vi "Main Loop.vi"(8 "error in (no error)":errorcluster, 10 "Chart Notifier":refnum<notifier>, 11 "Message Queues":T1) -> (0 "error out":errorcluster)   [LabVIEW 2018, in "Pump Module.lvlib" / "Pump Module Engine.lvlib"]
uses:
  Pump Module Engine.lvlib
  All Message Queues.ctl
  support/Message Queue/Message Cluster.ctl
  State Cluster.ctl
  State Enum.ctl
  Pump Module Settings Cluster.ctl
  Measure Instrument/PID 2 Output Enum.ctl
  Ismatec ISM 831C/Controls/Ismatech Settings Cluster.ctl
  Masterflex 7550-30/Controls/Settings Cluster.ctl
  VICI M50 Party Mode/Settings Cluster.ctl
  Tacmina QI/Tacmina QI DAQ Setting.ctl
  KNF Pump/Settings Cluster plus SIMDOS.ctl
  ASIA Pump/Pump Settings.ctl
  FLOM Pump/Settings Cluster.ctl
  SSI PR Class/SSI PR or LD Settings Cluster.ctl
  Masterflex 75211/Masterflex 75211 DAQ Setting.ctl
  Pump Module Display.ctl
  <vilib>/Platform/TimedLoop/XDataNode/timing_clust.ctl
  <vilib>/Platform/TimedLoop/XDataNode/nitl_modes.ctl
  <vilib>/Platform/TimedLoop/XDataNode/wakeup.ctl
  Tag VIs/Tag FGV Operation Enum.ctl
  support/Message Queue/Enqueue Message (Single).vi
  <vilib>/Platform/TimedLoop/XDataNode/XDataNode.xnode
  support/Message Queue/Message Queue.lvlib
  <vilib>/Platform/TimedLoop/XDataNode/XDNodeRunTimeDep.lvlib
  Pump Module.lvlib
  Ismatec ISM 831C/Ismatec ISM 831C.lvlib
  Masterflex 7550-30/Masterflex 7550-30.lvlib
  Shared Variables/Dynamic Shared Variables.lvlib
  Tacmina QI/Tacmina QI.lvlib
  KNF Pump/KNF SIMDOS.lvlib
  ASIA Pump.lvlib
  VICI M50 Party Mode/VICI M6 M50 Party Mode.lvlib
  FLOM Pump/FLOM Pump.lvlib
  SSI PR Class/SSI PR or LD Pump.lvlib
  support/Support Library.lvlib
  Masterflex 75211/Masterflex 75211.lvlib
panel:
  out "Period (s)":dbl format="%_4g"
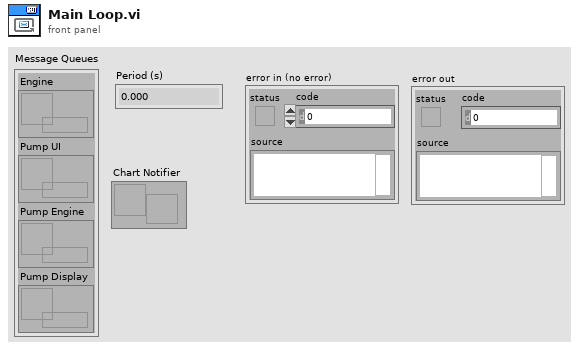
[diagram p1: front panel]
types:
  T1 = typedef "Pump Module.lvlib/All Message Queues.ctl" = cluster{"Engine":refnum<queue>, "Pump UI":refnum<queue>, "Pump Engine":refnum<queue>, "Pump Display":refnum<queue>}
  T2 = typedef "Pump Module.lvlib/Pump Module Display.ctl" = cluster{"Pump On?":enum16{"Off", "On", "Not Initialized"}, "Cycle Period":dbl, "Current Pump Speed":dbl, "Current Pump Pressure":dbl, "Current Pump Flow":dbl, "Output":T3}
  T3 = typedef "PID 2 Output Enum.ctl" = enum16{"Default", "Ismatec ISM 831C", "Masterflex 7550-30", "VICI", "Tacmina QI", "KNF SIMDOS", "ASIA Type C", "FLOM UI-22-11", "SSI PR/LD", "SSI P40", "Masterflex 75211-70"}
  T4 = typedef "XDNodeRunTimeDep.lvlib/timing_clust.ctl" = cluster{"Expected End [f-1]":u64, "Actual End [f-1]":u64, "Finished Late? [f-1]":bool, "Expected End [i-1]":u64, "Actual End [i-1]":u64, "Finished Late? [i-1]":bool, "Expected Start [i]":u64, "Actual Start [i]":u64, "Expected Start [f]":u64, "Actual Start [f]":u64, "Source Name":string, "Structure Name":string, "Period":i64, "Deadline":i64, "Offset":i64, "Start":i64, "Priority":i32, "Timeout":i32, "Mode":T5, "Wakeup Reason":T6, "Error":errorcluster, "Source Type":string, "Secondary Source Type":string, "Global End Time":u64, "Global Start Time":u64, "Frame Duration":u64, "Iteration Duration":u64, "Assigned CPU":i32, "I/O Scan Engine Mode":u32}
  T5 = typedef "XDNodeRunTimeDep.lvlib/nitl_modes.ctl" = enum32{"No Change", "Process missed periods, maintain original phase", "Discard missed periods, maintain original phase", "Process missed periods, ignore original phase", "Discard missed periods, ignore original phase"}
  T6 = typedef "XDNodeRunTimeDep.lvlib/wakeup.ctl" = enum32{"Normal", "Aborted", "Asynchronous wakeup", "Timing source error", "Timed loop error", "Timeout"}
  T7 = cluster{"enable? (F)":bool, "name":string, "alarm on":bool, "priority":u32, "ack type":enum16{"Auto", "User", "None", "Each Occurrence"}, "area":string, "description":string, "log? (T)":bool}
  T8 = typedef "Tag FGV Operation Enum.ctl" = enum16{"Init", "Set Notification Queue", "Create Tag", "Commit", "Write Tag (Numeric)", "Write Tag (Boolean)", "Read All Tags", "Read One Tag", "Delete Tag Category", "Set Alarm Parameters (Numeric)", "Set Alarm Parameters (Boolean)", "Enable All Alarms", "Disable All Alarms", "Delete All Tags", "Read Alarms", "Ack Alarm", "Read Alarm Parameters (Numeric)", "Read Alarm Parameters (Boolean)"}
  T9 = enum32{"u32BitField", "bool", "double", "string", "int8", "uint8", "int16", "uint16", "int32", "uint32", "int64", "uint64", "single", "double waveform", "int16 waveform", "array of boolean", "array of int8", "array of uint8", "array of int16", "array of uint16", "array of int32", "array of uint32", "array of int64", "array of uint64", "array of single", "array of double", "array of double waveform", "array of int16 waveform", "array of string", "variant", "timestamp", "fixed point", "custom"}
  T10 = typedef "Pump Module.lvlib/Pump Module Engine.lvlib/State Enum.ctl" = enum16{"Measuring", "Idle", "Paused"}
  T11 = typedef "Pump Module.lvlib/Pump Module Engine.lvlib/State Cluster.ctl" = cluster{"State":T10, "Start Time":timestamp, "Configuration":T12, "Current Time":timestamp, "First Iteration":bool, "Data":cluster{"Pump Speed":dbl, "Pump Pressure":dbl, "Pump Flow":dbl}, "Process Name":string, "Pump On?":enum16{"Off", "On", "Not Initialized"}, "Output Error":bool, "Log Started":bool, "Overpressure Alarming":bool}
  T12 = typedef "Pump Module.lvlib/Pump Module Settings Cluster.ctl" = cluster{"Cycle Period":dbl, "Manual Entry":dbl, "Output Device":T3, "Ismatech":T13, "Masterflex":T14, "VICI Settings":T15, "Tacmina Settings":T16, "KNF SIMDOS Settings":T17, "ASIA Pump C":T18, "FLOM Settings":T19, "SSI PR/LD Settings":T20, "SSI P40 Settings":T20, "Masterflex 75211 Settings":T21, "Pump Calibration File":path, "Calibration Slope":dbl, "Calibration Y Intercept":dbl, "Pump Cal Enum":u16}
  T13 = typedef "Ismatec ISM 831C.lvlib/Ismatech Settings Cluster.ctl" = cluster{"VISA resource name":refnum<visa-resource-name>, "Simulated?":bool, "Pump Number":dbl, "Reverse?":bool}
  T14 = typedef "Masterflex 7550-30.lvlib/Settings Cluster.ctl" = cluster{"VISA resource name":refnum<visa-resource-name>, "Simulated?":bool, "Pump Number":dbl, "Reverse?":bool}
  T15 = typedef "VICI M6 M50 Party Mode.lvlib/Settings Cluster.ctl" = cluster{"VISA resource name":refnum<visa-resource-name>, "Simulated?":bool, "Pump Letter":string, "Reverse?":bool}
  T16 = typedef "Tacmina QI.lvlib/Tacmina QI DAQ Setting.ctl" = cluster{"Analog DAQ Task":refnum<k21>, "Digital DAQ Task":refnum<k21>}
  T17 = typedef "KNF SIMDOS.lvlib/Settings Cluster plus SIMDOS.ctl" = cluster{"VISA resource name":refnum<visa-resource-name>, "Simulated?":bool}
  T18 = typedef "ASIA Pump.lvlib/Pump Settings.ctl" = cluster{"ASIA Pump #":i32, "channel":i32, "Simulated":bool}
  T19 = typedef "FLOM Pump.lvlib/Settings Cluster.ctl" = cluster{"VISA resource name":refnum<visa-resource-name>, "Simulated?":bool, "Pump Number":dbl}
  T20 = typedef "SSI PR or LD Pump.lvlib/SSI PR or LD Settings Cluster.ctl" = cluster{"VISA resource name":refnum<visa-resource-name>, "Simulated?":bool}
  T21 = typedef "Masterflex 75211.lvlib/Masterflex 75211 DAQ Setting.ctl" = cluster{"Analog DAQ Task":refnum<k21>, "Digital DAQ Task":refnum<k21>}
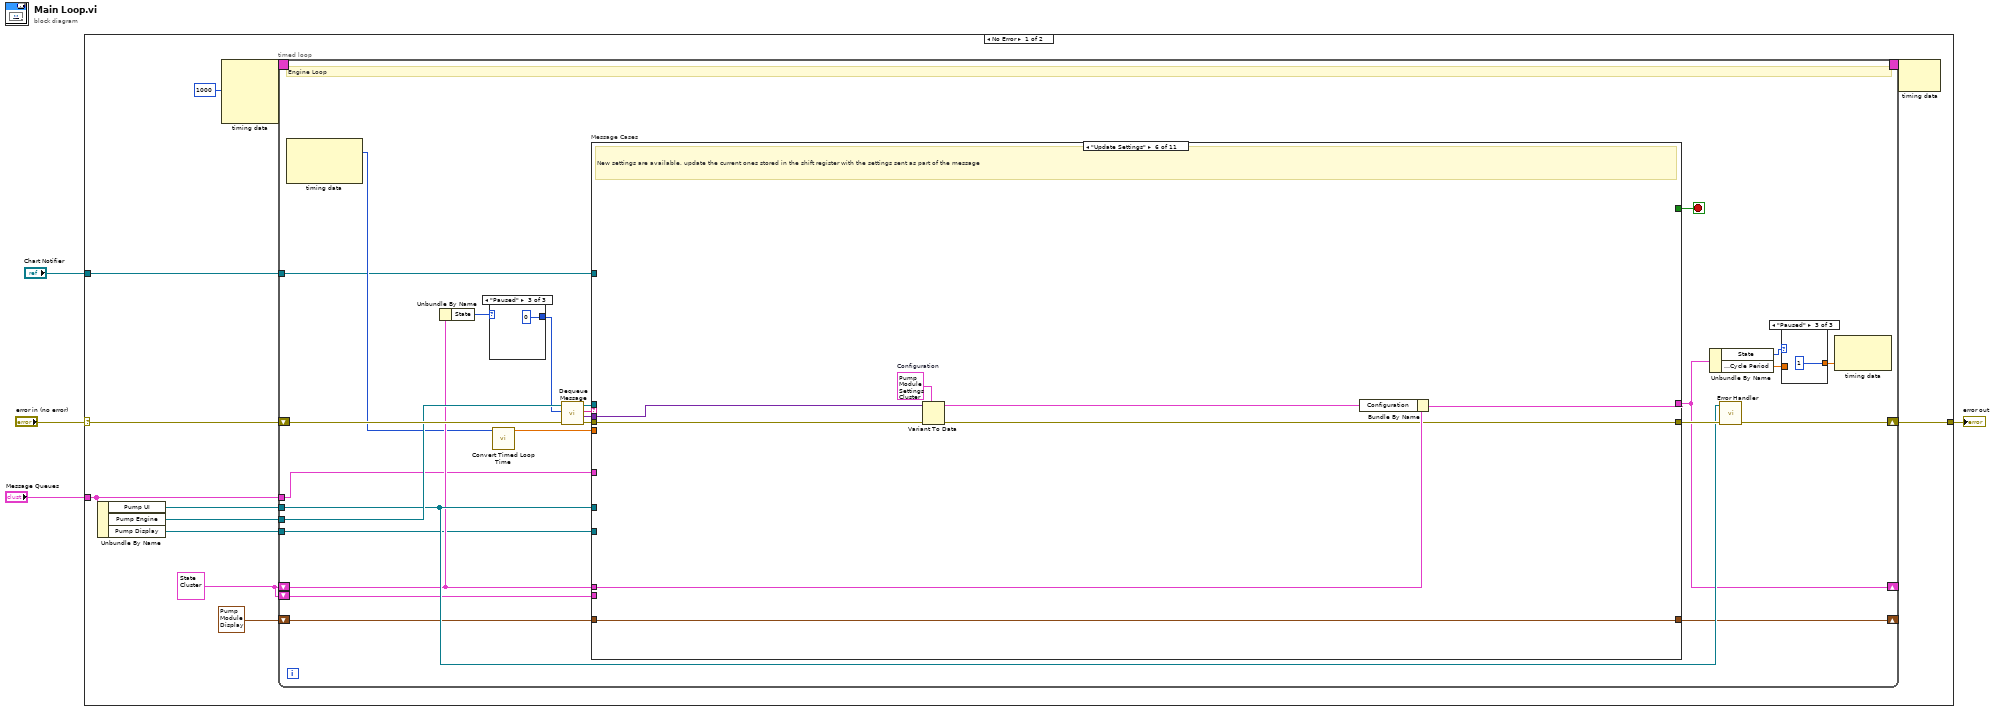
[diagram p0: block diagram]
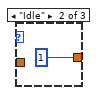
[diagram p3: hidden frame]
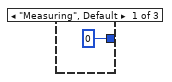
[diagram p4: hidden frame]
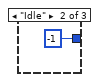
[diagram p5: hidden frame]
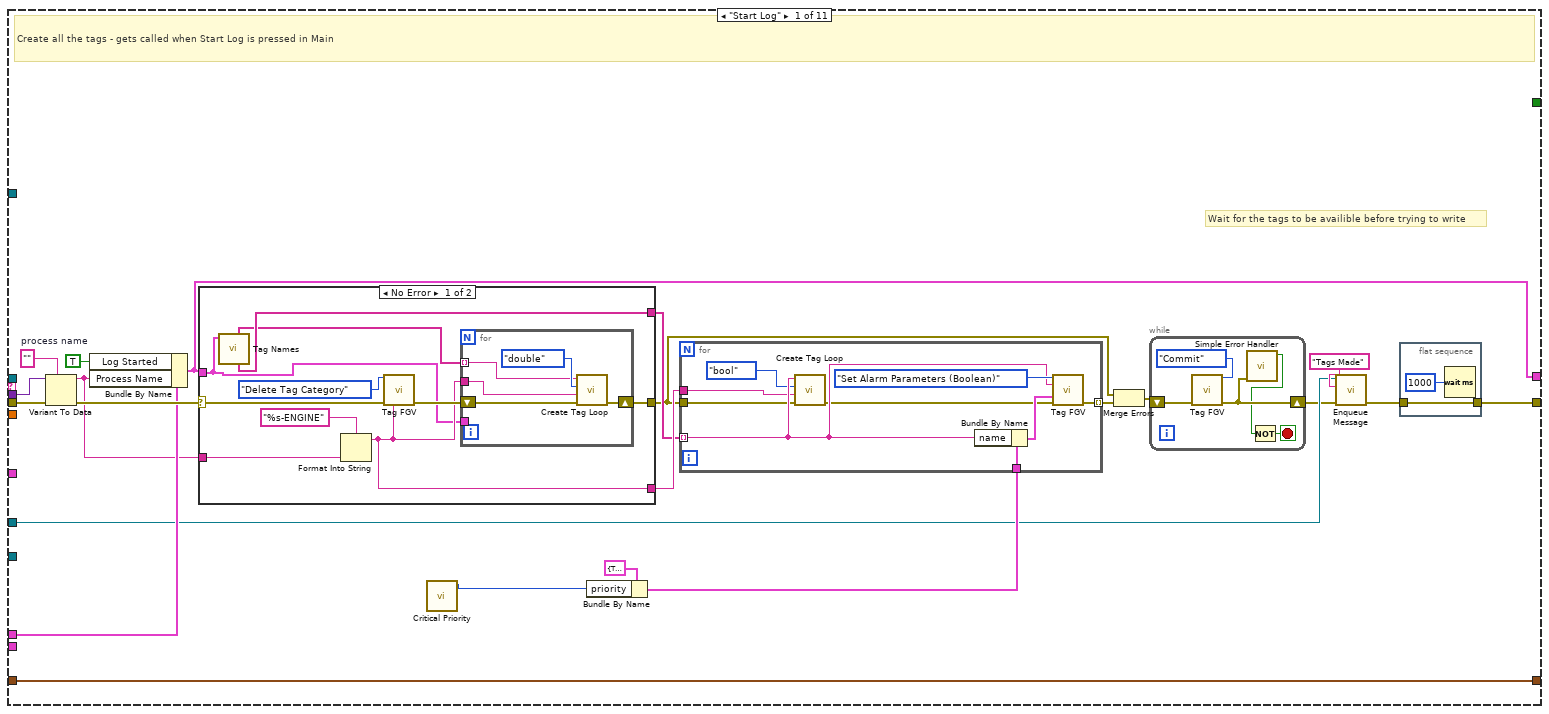
[diagram p6: hidden frame]
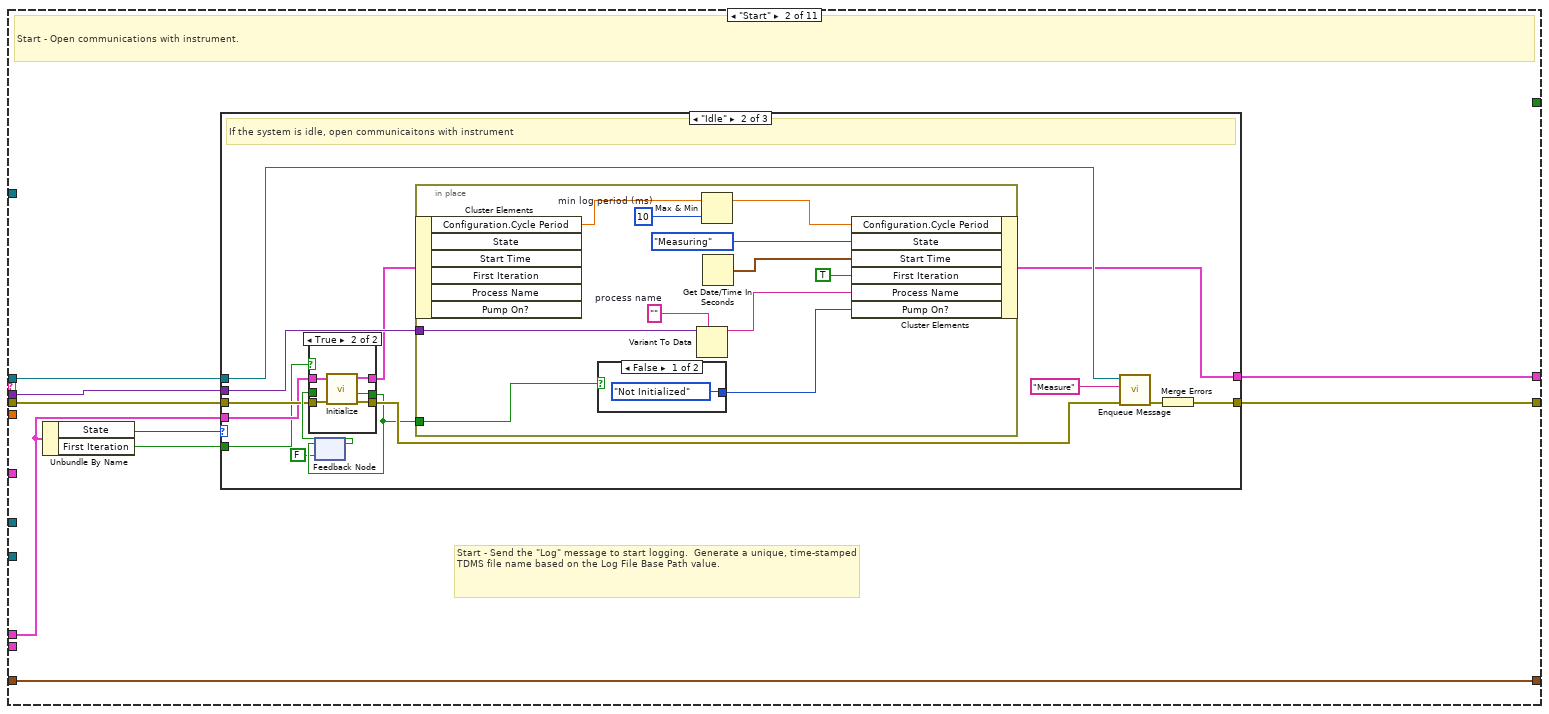
[diagram p8: hidden frame]
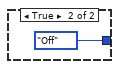
[diagram p10: hidden frame]
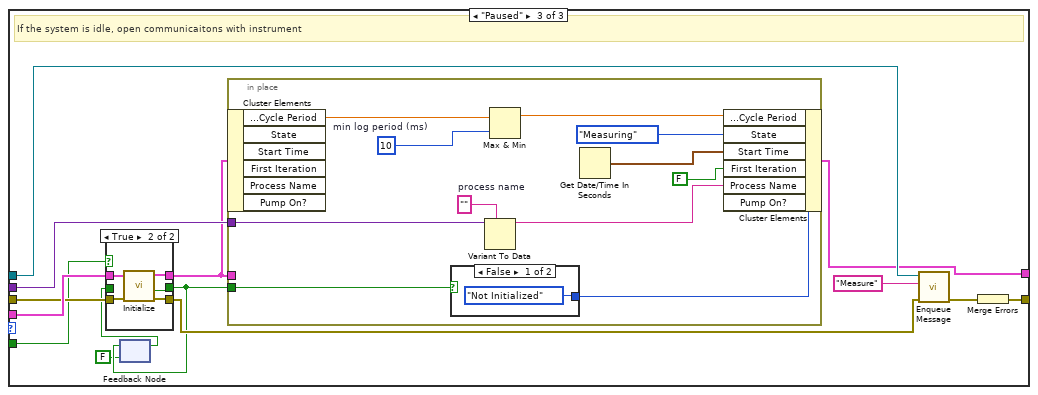
[diagram p12: hidden frame]
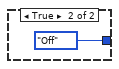
[diagram p13: hidden frame]
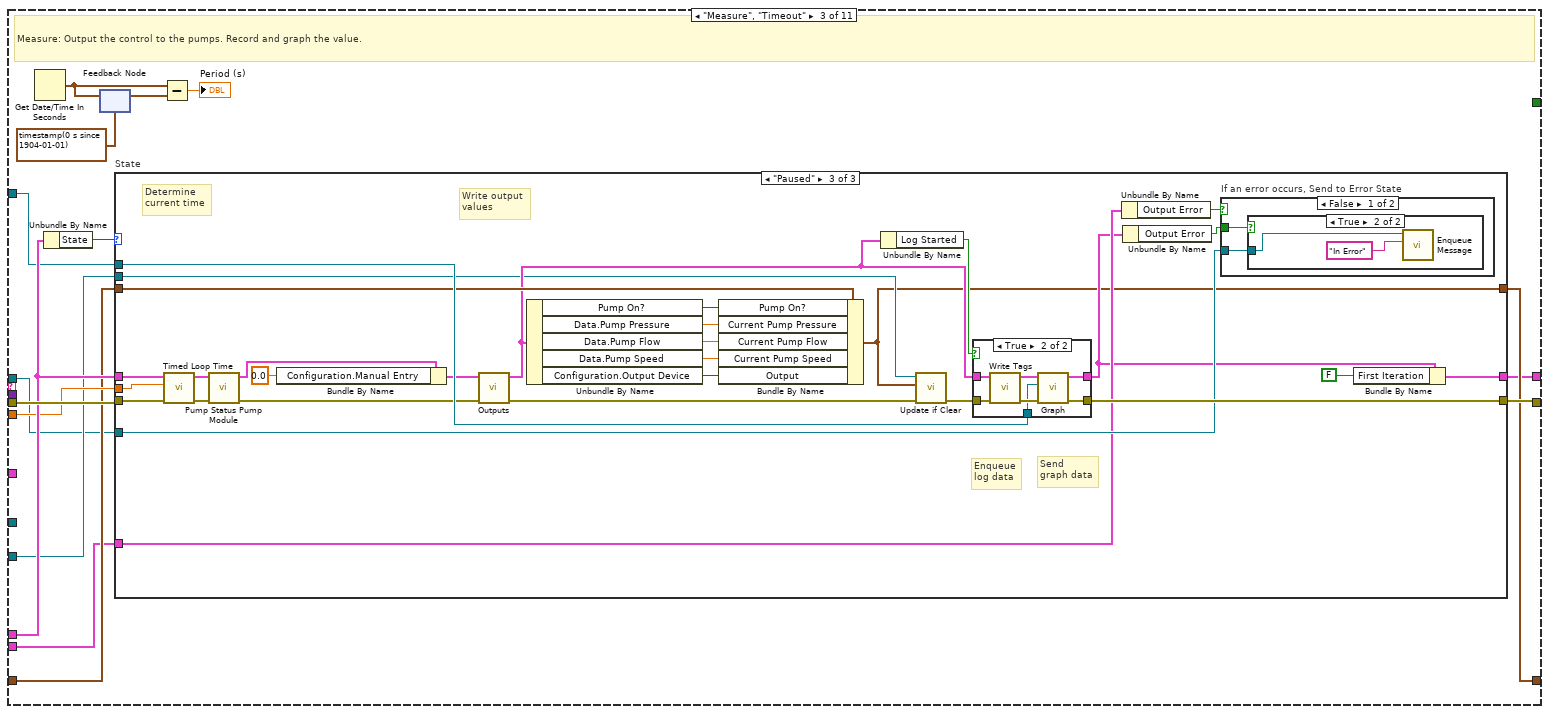
[diagram p15: hidden frame]
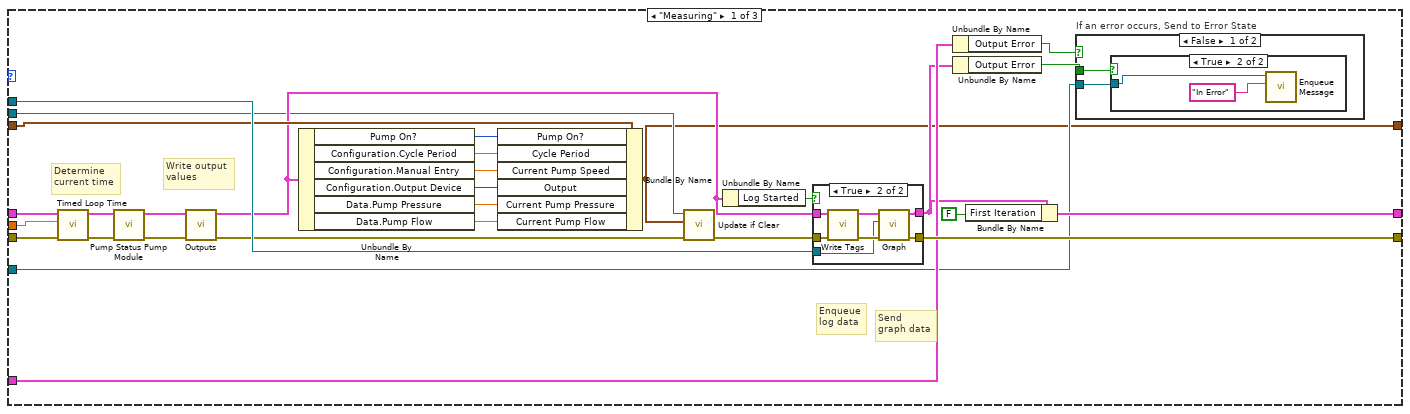
[diagram p16: hidden frame]
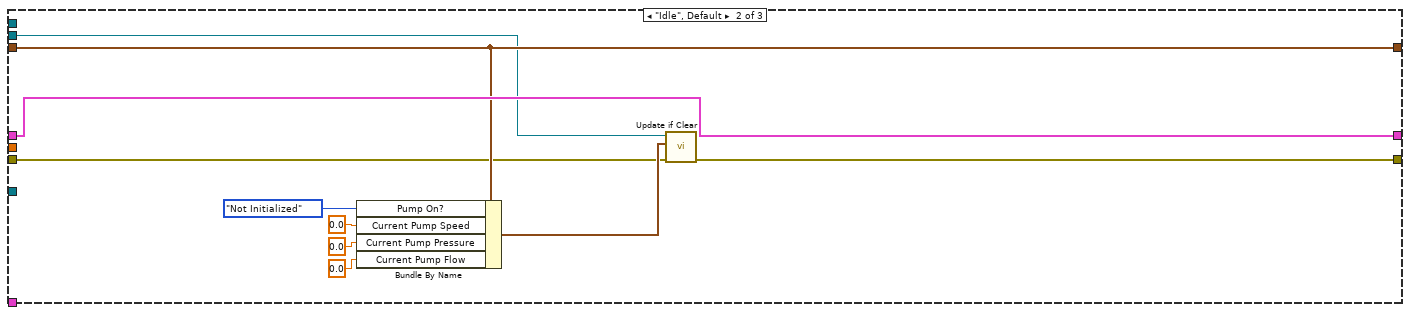
[diagram p20: hidden frame]
diagram:
  n1 = case shown="No Error" "error in (no error)" {
    selector: "error in (no error)" -> [w15 w430]
    tunnel: "Message Queues" -> [w11 _]
    tunnel: [w16 w430] -> w3
    tunnel: "Chart Notifier" -> [w9 _]
    frame No Error {
      w6 = T11 {"State"=enum."Idle", "Start Time"=timestamp(0 s since 1904-01-01), "Configuration"={"Cycle Period"=0.0, "Manual Entry"=0.0, "Output Device"=enum."VICI", "Ismatech"={"VISA resource name"="", "Simulated?"=FALSE, "Pump Number"=1.0, "Reverse?"=FALSE}, "Masterflex"={"VISA resource name"="", "Simulated?"=FALSE, "Pump Number"=1.0, "Reverse?"=FALSE}, "VICI Settings"={"VISA resource name"="", "Simulated?"=FALSE, "Pump Letter"="", "Reverse?"=FALSE}, "Tacmina Settings"={"Analog DAQ Task"="", "Digital DAQ Task"=""}, "KNF SIMDOS Settings"={"VISA resource name"="", "Simulated?"=TRUE}, "ASIA Pump C"={"ASIA Pump #"=0, "channel"=0, "Simulated"=FALSE}, "FLOM Settings"={"VISA resource name"="", "Simulated?"=TRUE, "Pump Number"=0.0}, "SSI PR/LD Settings"={"VISA resource name"="", "Simulated?"=FALSE}, "SSI P40 Settings"={"VISA resource name"="", "Simulated?"=FALSE}, "Masterflex 75211 Settings"={"Analog DAQ Task"="", "Digital DAQ Task"=""}, "Pump Calibration File"=path "", "Calibration Slope"=0.0, "Calibration Y Intercept"=0.0, "Pump Cal Enum"=0}, "Current Time"=timestamp(0 s since 1904-01-01), "First Iteration"=FALSE, "Data"={"Pump Speed"=0.0, "Pump Pressure"=0.0, "Pump Flow"=0.0}, "Process Name"="", "Pump On?"=enum."Off", "Output Error"=FALSE, "Log Started"=FALSE, "Overpressure Alarming"=FALSE}
      n2 = Unbundle By Name(w11) -> ("Pump UI"=w14:refnum<queue>, "Pump Engine"=w10:refnum<queue>, "Pump Display"=w8:refnum<queue>)
      n3 = node-c288(i64 1000 ("Period")) -> (w13:T4)  [unwired: 3 in]
      n4 = timed-loop {
        tunnel: w10 -> [w35]
        shift-right: [w17] -> _
        shift-left: w6 -> [w31]
        shift-right: [w33] -> w16
        shift-left: w15 -> [w40]
        tunnel: w14 -> [w32]
        timing: w13 -> [_]
        timing-out: [_] -> w12
        tunnel: w11 -> [w23]
        tunnel: w9 -> [w22]
        tunnel: w8 -> [w21]
        shift-right: [w20] -> _
        shift-left: T2 {"Pump On?"=enum."Off", "Cycle Period"=500.0, "Current Pump Speed"=0.0, "Current Pump Pressure"=0.0, "Current Pump Flow"=0.0, "Output"=enum."Default"} ("PM Display") -> [w19]
        shift-left: w6 -> [w18]
        stop <- w41 stop-if-true
        # "Engine Loop"
        n5 = node-c288() -> (w25:i64)  [unwired: 1 in, 2 out]
        n6 = Unbundle By Name(w31) -> ("State"=w30:T10)
        n7 = case shown="\"Paused\"" w30 {
          tunnel: [0 ("timeout in ms (-1)") -1 ("timeout in ms (-1)") 0 ("timeout in ms (-1)")] -> w29
          frame "Measuring", Default {
          }
          frame "Idle" {
          }
          frame "Paused" {
          }
        }
        n8 = call "Convert Timed Loop Time.vi"("Actual Start [i]"=w25) -> ("ET since start (s)"=w24:dbl)  [unwired: 10 in]
        n9 = call "Dequeue Message.vi"("error in (no error)"=w40, "timeout in ms (-1)"=w29, "Message Queue"=w35) -> ("error out"=w39:errorcluster, "Message Data"=w37:variant, "Message"=w38:string, "dup Message Queue"=w36:refnum<queue>)  [unwired: 5 in]
        n10 = case "Message Cases" shown="\"Update Settings\"" w38 {
          selector: w38 -> [_ _ _ _ _ _ _ _ _ _ w419]
          tunnel: w36 -> [_ w114 w191 _ _ _ w370 _ w385 _ _]
          tunnel: w39 -> [w58 w113 w201 w304 w326 w364 w373 w380 w399 w417 _]
          tunnel: [w54 w115 w202 w299 w320 w360 w375 w379 w394 w416 w418] -> w34
          tunnel: w31 -> [w64 w110 w200 w306 w327 w361 w366 w377 w398 w414 w424]
          tunnel: [w60 w107 w189 w305 w329 w359 w366 w377 w395 w412 w424] -> w17
          tunnel: [_ _ _ _ _ _ TRUE _ _ _ _] -> w41
          tunnel: w37 -> [w73 w111 _ _ _ w365 _ _ _ _ _]
          tunnel: w32 -> [w61 _ _ w308 _ _ w374 _ _ _ _]
          tunnel: w24 -> [_ _ w199 _ _ _ _ _ _ _ _]
          tunnel: w23 -> [_ _ _ _ _ _ _ _ _ _ _]
          tunnel: w22 -> [_ _ w195 _ _ _ _ _ _ _ _]
          tunnel: w21 -> [_ _ w194 w302 w323 _ _ _ w384 _ _]
          tunnel: w19 -> [w74 w109 w193 w301 w322 w362 w367 w378 w392 w415 w425]
          tunnel: [w74 w109 w192 w301 w322 w362 w367 w378 w383 w415 w425] -> w20
          tunnel: w18 -> [_ _ w190 _ _ _ _ _ _ _ _]
          frame "Start Log" {
            w72 = ""  # process name
            # "Wait for the tags to be availible before trying to write"
            # "Create all the tags - gets called when Start Log is pressed in Main"
            n11 = Variant To Data(error in=w58, type=w72, Variant=w73) -> (data=w59:string, error out=w71:errorcluster)
            n12 = Bundle By Name(cluster=w64, "Log Started"=TRUE, "Process Name"=w59) -> (w60:T11)
            n13 = case shown="No Error" w71 {
              selector: w71 -> [w97 w106]
              tunnel: [w100 w106] -> w53
              tunnel: [w95 _] -> w67
              tunnel: [w94 _] -> w66
              tunnel: w60 -> [w91 _]
              tunnel: w59 -> [w93 _]
              frame No Error {
                n14 = call "Tag Names.vi"("State In"=w91) -> ("All Boolean Tags"=w94:string[], "All  Numeric Tags"=w92:string[])  [unwired: 8 in, 1 out]
                n15 = Format Into String(format string="%s-ENGINE", w93) -> (resulting string=w95:string)  [unwired: 2 in, 1 out]
                n16 = call "Tag FGV.vi"("Operation"=Tag_FGV_Operation_Enum."Delete Tag Category", "error in (no error)"=w97, "Tag Category"=w95) -> ("error out"=w96:errorcluster)  [unwired: 5 in, 7 out]
                n17 = for {
                  shift-right: [w101] -> w100
                  shift-left: w96 -> [w102]
                  tunnel: w95 -> [w103]
                  tunnel: w92 -> [w104] mode=indexing
                  tunnel: w91 -> [_]
                  n18 = call "Create Tag Loop.vi"("error in (no error)"=w102, "Tag Category"=w103, "data type"=T9."double", "Tag Name"=w104) -> ("error out"=w101:errorcluster)  [unwired: 7 in]
                }
              }
              frame Error {
              }
            }
            n19 = call "Critical Priority.vi"() -> ("critical priority"=w70:i32)  [unwired: 11 in]
            n20 = Bundle By Name(cluster=T7 {"enable? (F)"=TRUE, "name"="Boolean", "alarm on"=TRUE, "priority"=1, "ack type"=enum."Each Occurrence", "area"="a", "description"="", "log? (T)"=TRUE} ("Boolean alarm settings"), "priority"=w70) -> (w68:T7)
            n21 = for {
              tunnel: w68 -> [w90]
              tunnel: [w89] -> w65 mode=indexing
              tunnel: w66 -> [w86] mode=indexing
              tunnel: w53 -> [w83]
              tunnel: w67 -> [w84]
              n22 = call "Create Tag Loop.vi"("error in (no error)"=w83, "Tag Category"=w84, "data type"=T9."bool", "Tag Name"=w86) -> ("error out"=w82:errorcluster)  [unwired: 7 in]
              n23 = Bundle By Name(cluster=w90, "name"=w86) -> (w88:T7)
              n24 = call "Tag FGV.vi"("Operation"=Tag_FGV_Operation_Enum."Set Alarm Parameters (Boolean)", "Tag Name"=w86, "Data"=w88, "error in (no error)"=w82) -> ("error out"=w89:errorcluster)  [unwired: 4 in, 7 out]
            }
            n25 = Merge Errors(w53, w65) -> (w57:errorcluster)
            n26 = while {
              shift-right: [w79] -> w56
              shift-left: w57 -> [w80]
              stop <- w77 stop-if-true
              n27 = call "Tag FGV.vi"("Operation"=Tag_FGV_Operation_Enum."Commit", "error in (no error)"=w80) -> ("error out"=w79:errorcluster)  [unwired: 6 in, 7 out]
              n28 = call <vilib>:"Simple Error Handler.vi"("error in (no error)"=w79) -> ("error?"=w78:bool)  [unwired: 4 in, 4 out]
              n29 = Not(x=w78) -> (.not. x?=w77:bool)
            }
            n30 = call-poly "Enqueue Message.vi"("error in (no error)"=w56, "Message"="Tags Made", "Message Queue"=w61) -> ("error out"=w55:errorcluster)  [unwired: 7 in, 1 out]
            n31 = flat-sequence {
              tunnel: [w75] -> w54
              tunnel: w55 -> [w75]
              frame #0 {
                n32 = Wait (ms)(milliseconds to wait=u32 1000) -> ()  [unwired: 1 out]
              }
            }
          }
          frame "Start" {
            # "Start - Send the \"Log\" message to start logging.  Generate a unique, time-stamped TDMS file name based on the Log File Base Path value."
            # "Start - Open communications with instrument."
            n33 = Unbundle By Name(w110) -> ("State"=w112:T10, "First Iteration"=w108:bool)
            n34 = case shown="\"Idle\"" w112 {
              tunnel: [w116 w131 w166] -> w115
              tunnel: w114 -> [_ w128 w163]
              tunnel: w113 -> [w116 w125 w160]
              tunnel: w110 -> [w117 w124 w161]
              tunnel: [w117 w119 w154] -> w107
              tunnel: w111 -> [_ w127 w162]
              tunnel: w108 -> [_ w121 w156]
              frame "Measuring", Default {
                # "The system is already running. Ignore the \"Start\" message."
              }
              frame "Idle" {
                # "If the system is idle, open communicaitons with instrument"
                n35 = feedback #1(FALSE ("Initialized")) -> (w126:bool)
                n36 = case shown="True" w121 {
                  tunnel: w125 -> [w146 w151]
                  tunnel: w124 -> [w147 w152]
                  tunnel: [w147 w150] -> w120
                  tunnel: [w146 w148] -> w123
                  tunnel: [w145 w149] -> w122
                  tunnel: w126 -> [w145 _]
                  frame False {
                  }
                  frame True {
                    n37 = call "Initialize.vi"("error in (no error)"=w151, "State in"=w152) -> ("error out"=w148:errorcluster, "Initialized"=w149:bool, "State out"=w150:T11)  [unwired: 7 in]
                  }
                }
                n38 = feedback-in #1(w122) -> ()
                n39 = in-place {
                  in-place-border: w127 -> [w140]
                  in-place-border: w122 -> [w139]
                  w141 = ""  # process name
                  w142 = 10  # min log period (ms)
                  n40 = in-place-cluster #2(w120) -> ("Configuration.Cycle Period"=w138:dbl)  [unwired: 5 out]
                  n41 = case shown="False" w139 {
                    tunnel: [enum16{"Off", "On", "Not Initialized"}."Not Initialized" ("Pump On?") enum16{"Off", "On", "Not Initialized"}."Off" ("Pump On?")] -> w132
                    frame False {
                    }
                    frame True {
                    }
                  }
                  n42 = Variant To Data(type=w141, Variant=w140) -> (data=w133:string)  [unwired: 1 in, 1 out]
                  n43 = Max & Min(x=w138, y=w142) -> (max(x,y)=w137:dbl)  [unwired: 1 out]
                  n44 = Get Date/Time In Seconds() -> (seconds since 1Jan1904=w135:timestamp)
                  n45 = in-place-cluster #2("Configuration.Cycle Period"=w137, "State"=State_Enum."Measuring", "Start Time"=w135, "First Iteration"=TRUE, "Process Name"=w133, "Pump On?"=w132) -> (w119:T11)
                }
                n46 = call-poly "Enqueue Message.vi"("error in (no error)"=w123, "Message"="Measure", "Message Queue"=w128) -> ("error out"=w129:errorcluster)  [unwired: 7 in, 1 out]
                n47 = Merge Errors(w129) -> (w131:errorcluster)
              }
              frame "Paused" {
                # "If the system is idle, open communicaitons with instrument"
                n48 = feedback #3(FALSE ("Initialized")) -> (w157:bool)
                n49 = case shown="True" w156 {
                  tunnel: w160 -> [w181 w186]
                  tunnel: w161 -> [w182 w187]
                  tunnel: [w182 w185] -> w155
                  tunnel: [w181 w183] -> w159
                  tunnel: [w180 w184] -> w158
                  tunnel: w157 -> [w180 _]
                  frame False {
                  }
                  frame True {
                    n50 = call "Initialize.vi"("error in (no error)"=w186, "State in"=w187) -> ("error out"=w183:errorcluster, "Initialized"=w184:bool, "State out"=w185:T11)  [unwired: 7 in]
                  }
                }
                n51 = feedback-in #3(w158) -> ()
                n52 = in-place {
                  in-place-border: w162 -> [w175]
                  in-place-border: w155 -> [_]
                  in-place-border: w158 -> [w174]
                  w176 = ""  # process name
                  w177 = 10  # min log period (ms)
                  n53 = in-place-cluster #4(w155) -> ("Configuration.Cycle Period"=w173:dbl)  [unwired: 5 out]
                  n54 = case shown="False" w174 {
                    tunnel: [enum16{"Off", "On", "Not Initialized"}."Not Initialized" ("Pump On?") enum16{"Off", "On", "Not Initialized"}."Off" ("Pump On?")] -> w167
                    frame False {
                    }
                    frame True {
                    }
                  }
                  n55 = Variant To Data(type=w176, Variant=w175) -> (data=w168:string)  [unwired: 1 in, 1 out]
                  n56 = Max & Min(x=w173, y=w177) -> (max(x,y)=w172:dbl)  [unwired: 1 out]
                  n57 = Get Date/Time In Seconds() -> (seconds since 1Jan1904=w170:timestamp)
                  n58 = in-place-cluster #4("Configuration.Cycle Period"=w172, "State"=State_Enum."Measuring", "Start Time"=w170, "First Iteration"=FALSE, "Process Name"=w168, "Pump On?"=w167) -> (w154:T11)
                }
                n59 = call-poly "Enqueue Message.vi"("error in (no error)"=w159, "Message"="Measure", "Message Queue"=w163) -> ("error out"=w164:errorcluster)  [unwired: 7 in, 1 out]
                n60 = Merge Errors(w164) -> (w166:errorcluster)
              }
            }
          }
          frame "Measure", "Timeout" {
            # "Measure: Output the control to the pumps. Record and graph the value."
            n61 = Get Date/Time In Seconds() -> (seconds since 1Jan1904=w197:timestamp)
            n62 = Unbundle By Name(w200) -> ("State"=w203:T10)
            n63 = feedback-in #5(w197) -> ()
            n64 = feedback #5(timestamp(0 s since 1904-01-01) ("seconds since 1Jan1904")) -> (w198:timestamp)
            n65 = case "State" shown="\"Paused\"" w203 {
              tunnel: w201 -> [w231 w247 w279]
              tunnel: w200 -> [w230 w255 w280]
              tunnel: [w232 w246 w274] -> w202
              tunnel: [w228 w255 w264] -> w189
              tunnel: w199 -> [w229 _ w284]
              tunnel: w195 -> [w226 _ w285]
              tunnel: w194 -> [w207 w249 w259]
              tunnel: w193 -> [w223 w254 w283]
              tunnel: [w206 w254 w258] -> w192
              tunnel: w191 -> [w211 _ w270]
              tunnel: w190 -> [w213 _ w268]
              frame "Measuring" {
                # "Determine\ncurrent time"
                # "Send\ngraph data"
                # "Enqueue\nlog data"
                # "Write output\nvalues"
                n66 = call "Timed Loop Time.vi"("error in (no error)"=w231, "ET since start (s)"=w229, "State in"=w230) -> ("error out"=w221:errorcluster, "State out"=w220:T11)  [unwired: 7 in]
                n67 = call "Pump Status Pump Module.vi"("error in (no error)"=w221, 11:w220) -> ("error out"=w224:errorcluster, "State out"=w225:T11)  [unwired: 8 in]
                n68 = call "Outputs.vi"("error in (no error)"=w224, "State in"=w225) -> ("error out"=w205:errorcluster, "State out"=w217:T11)  [unwired: 8 in]
                n69 = Unbundle By Name(w217) -> ("Pump On?"=w222:enum16{"Off", "On", "Not Initialized"}, "Configuration.Cycle Period"=w219:dbl, "Configuration.Manual Entry"=w218:dbl, "Configuration.Output Device"=w210:T3, "Data.Pump Pressure"=w209:dbl, "Data.Pump Flow"=w208:dbl)
                n70 = Bundle By Name(cluster=w223, "Pump On?"=w222, "Cycle Period"=w219, "Current Pump Speed"=w218, "Output"=w210, "Current Pump Pressure"=w209, "Current Pump Flow"=w208) -> (w206:T2)
                n71 = call "Update if Clear.vi"("error in (no error)"=w205, "Message Data"=w206, "Queue in"=w207) -> ("error out"=w204:errorcluster)  [unwired: 8 in]
                n72 = Unbundle By Name(w217) -> ("Log Started"=w216:bool)
                n73 = case shown="True" w216 {
                  tunnel: [w237 w243] -> w232
                  tunnel: [w238 w242] -> w212
                  tunnel: w226 -> [_ w241]
                  tunnel: w217 -> [w238 w240]
                  tunnel: w204 -> [w237 w239]
                  frame False {
                  }
                  frame True {
                    n74 = call "Write Tags.vi"("error in (no error)"=w239, "State in"=w240) -> ("error out"=w244:errorcluster, "State out"=w245:T11)  [unwired: 8 in]
                    n75 = call "Graph.vi"("error in (no error)"=w244, "notifier out"=w241, "State in"=w245) -> ("error out"=w243:errorcluster, "State out"=w242:T11)  [unwired: 7 in]
                  }
                }
                n76 = Unbundle By Name(w213) -> ("Output Error"=w214:bool)
                n77 = Unbundle By Name(w212) -> ("Output Error"=w215:bool)
                n78 = Bundle By Name(cluster=w212, "First Iteration"=FALSE) -> (w228:T11)
                n79 = case "If an error occurs, Send to Error State" shown="False" w214 {
                  tunnel: w215 -> [w234 _]
                  tunnel: w211 -> [w233 _]
                  frame False {
                    n80 = case shown="True" w234 {
                      tunnel: w233 -> [_ w235]
                      frame False {
                      }
                      frame True {
                        n81 = call-poly "Enqueue Message.vi"("Message"="In Error", "Message Queue"=w235) -> ()  [unwired: 8 in, 2 out]
                      }
                    }
                  }
                  frame True {
                  }
                }
              }
              frame "Idle", Default {
                n82 = Bundle By Name(cluster=w254, "Pump On?"=enum16{"Off", "On", "Not Initialized"}."Not Initialized", "Current Pump Speed"=0.0, "Current Pump Pressure"=0.0, "Current Pump Flow"=0.0) -> (w248:T2)
                n83 = call "Update if Clear.vi"("error in (no error)"=w247, "Message Data"=w248, "Queue in"=w249) -> ("error out"=w246:errorcluster)  [unwired: 8 in]
              }
              frame "Paused" {
                # "Determine\ncurrent time"
                # "Write output\nvalues"
                # "Send\ngraph data"
                # "Enqueue\nlog data"
                n84 = call "Timed Loop Time.vi"("error in (no error)"=w279, "ET since start (s)"=w284, "State in"=w280) -> ("error out"=w276:errorcluster, "State out"=w278:T11)  [unwired: 7 in]
                n85 = call "Pump Status Pump Module.vi"("error in (no error)"=w276, 11:w278) -> ("error out"=w275:errorcluster, "State out"=w277:T11)  [unwired: 8 in]
                n86 = Bundle By Name(cluster=w277, "Configuration.Manual Entry"=0.0) -> (w281:T11)
                n87 = call "Outputs.vi"("error in (no error)"=w275, "State in"=w281) -> ("error out"=w257:errorcluster, "State out"=w263:T11)  [unwired: 8 in]
                n88 = Unbundle By Name(w263) -> ("Pump On?"=w273:enum16{"Off", "On", "Not Initialized"}, "Data.Pump Pressure"=w272:dbl, "Data.Pump Flow"=w271:dbl, "Data.Pump Speed"=w261:dbl, "Configuration.Output Device"=w260:T3)
                n89 = Bundle By Name(cluster=w283, "Pump On?"=w273, "Current Pump Pressure"=w272, "Current Pump Flow"=w271, "Current Pump Speed"=w261, "Output"=w260) -> (w258:T2)
                n90 = Unbundle By Name(w263) -> ("Log Started"=w262:bool)
                n91 = call "Update if Clear.vi"("error in (no error)"=w257, "Message Data"=w258, "Queue in"=w259) -> ("error out"=w256:errorcluster)  [unwired: 8 in]
                n92 = case shown="True" w262 {
                  tunnel: w285 -> [_ w292]
                  tunnel: w256 -> [w286 w291]
                  tunnel: [w286 w290] -> w274
                  tunnel: w263 -> [w287 w289]
                  tunnel: [w287 w288] -> w265
                  frame False {
                  }
                  frame True {
                    n93 = call "Write Tags.vi"("error in (no error)"=w291, "State in"=w289) -> ("error out"=w294:errorcluster, "State out"=w293:T11)  [unwired: 8 in]
                    n94 = call "Graph.vi"("error in (no error)"=w294, "notifier out"=w292, "State in"=w293) -> ("error out"=w290:errorcluster, "State out"=w288:T11)  [unwired: 7 in]
                  }
                }
                n95 = Unbundle By Name(w268) -> ("Output Error"=w267:bool)
                n96 = Unbundle By Name(w265) -> ("Output Error"=w269:bool)
                n97 = case "If an error occurs, Send to Error State" shown="False" w267 {
                  tunnel: w269 -> [w296 _]
                  tunnel: w270 -> [w295 _]
                  frame False {
                    n98 = case shown="True" w296 {
                      tunnel: w295 -> [_ w298]
                      frame False {
                      }
                      frame True {
                        n99 = call-poly "Enqueue Message.vi"("Message"="In Error", "Message Queue"=w298) -> ()  [unwired: 8 in, 2 out]
                      }
                    }
                  }
                  frame True {
                  }
                }
                n100 = Bundle By Name(cluster=w265, "First Iteration"=FALSE) -> (w264:T11)
              }
            }
            n101 = Subtract(x=w197, y=w198) -> (x-y=→"Period (s)":dbl)
          }
          frame "Stop" {
            # "Stop - Flush the message queue of any pending \"Log\" messages. Call 'Flush Data to Log File.vi' so any pending data is not lost."
            n102 = call <vilib>:"Clear Errors.vi"("error in (no error)"=w304) -> ("error out"=w303:errorcluster)  [unwired: 5 in, 1 out]
            n103 = Unbundle By Name(w306) -> ("State"=w307:T10)
            n104 = case shown="\"Measuring\", Default" w307 {
              tunnel: [w313 w319] -> w300
              tunnel: w303 -> [w310 w319]
              tunnel: w308 -> [w317 _]
              tunnel: w306 -> [w311 w318]
              tunnel: [w315 w318] -> w305
              frame "Measuring", Default {
                # "If the system is logging, stop logging."
                n105 = call "Close.vi"("error in (no error)"=w310, "State in"=w311) -> ("error out"=w309:errorcluster, "State out"=w312:T11)  [unwired: 7 in, 1 out]
                n106 = Bundle By Name(cluster=w312, "State"=State_Enum."Idle") -> (w315:T11)
                n107 = call-poly "Enqueue Message.vi"("error in (no error)"=w309, "Message"="Logging Stopped", "Message Queue"=w317) -> ("error out"=w313:errorcluster)  [unwired: 7 in, 1 out]
              }
              frame "Idle" {
                # "The system is already idle. Ignore the \"Stop\" message."
              }
            }
            n108 = call "Update if Clear.vi"("error in (no error)"=w300, "Message Data"=w301, "Queue in"=w302) -> ("error out"=w299:errorcluster)  [unwired: 8 in]
          }
          frame "Pause" {
            # "Stop - Flush the message queue of any pending \"Log\" messages. Call 'Flush Data to Log File.vi' so any pending data is not lost."
            n109 = Unbundle By Name(w327) -> ("State"=w330:T10, "First Iteration"=w328:bool)
            n110 = case shown="True" w328 {
              tunnel: w327 -> [w331 w335]
              tunnel: [w331 w339] -> w325
              tunnel: w326 -> [w332 w336]
              tunnel: [w332 w337] -> w324
              frame False {
              }
              frame True {
                # "If we start on a pause condition, initialize the pump"
                n111 = call "Initialize.vi"("error in (no error)"=w336, "State in"=w335) -> ("error out"=w337:errorcluster, "Initialized"=w338:bool, "State out"=w334:T11)  [unwired: 7 in]
                n112 = case shown="True" w338 {
                  tunnel: [enum16{"Off", "On", "Not Initialized"}."Not Initialized" ("Pump On?") enum16{"Off", "On", "Not Initialized"}."Off" ("Pump On?")] -> w340
                  tunnel: [_ FALSE] -> w333
                  frame False {
                  }
                  frame True {
                  }
                }
                n113 = Bundle By Name(cluster=w334, "Pump On?"=w340, "First Iteration"=w333) -> (w339:T11)
              }
            }
            n114 = case shown="\"Measuring\", Default" w330 {
              tunnel: [w344 w353 w357] -> w321
              tunnel: w324 -> [w348 w353 w357]
              tunnel: w325 -> [w345 w351 w355]
              tunnel: [w346 w350 w354] -> w329
              frame "Measuring", Default {
                # "If the system is logging, stop logging."
                n115 = call "Pause.vi"("error in (no error)"=w348, "State in"=w345) -> ("error out"=w344:errorcluster, "State out"=w347:T11)  [unwired: 8 in]
                n116 = Bundle By Name(cluster=w347, "State"=State_Enum."Paused") -> (w346:T11)
              }
              frame "Idle" {
                # "The system is already idle. Ignore the \"Stop\" message."
                n117 = Bundle By Name(cluster=w351, "State"=State_Enum."Paused") -> (w350:T11)
              }
              frame "Paused" {
                n118 = Bundle By Name(cluster=w355, "State"=State_Enum."Paused") -> (w354:T11)
              }
            }
            n119 = call "Update if Clear.vi"("error in (no error)"=w321, "Message Data"=w322, "Queue in"=w323) -> ("error out"=w320:errorcluster)  [unwired: 8 in]
          }
          frame "Update Settings" {
            w363 = T12 {"Cycle Period"=0.0, "Manual Entry"=0.0, "Output Device"=enum."VICI", "Ismatech"={"VISA resource name"="", "Simulated?"=FALSE, "Pump Number"=1.0, "Reverse?"=FALSE}, "Masterflex"={"VISA resource name"="", "Simulated?"=FALSE, "Pump Number"=1.0, "Reverse?"=FALSE}, "VICI Settings"={"VISA resource name"="", "Simulated?"=FALSE, "Pump Letter"="", "Reverse?"=FALSE}, "Tacmina Settings"={"Analog DAQ Task"="", "Digital DAQ Task"=""}, "KNF SIMDOS Settings"={"VISA resource name"="", "Simulated?"=TRUE}, "ASIA Pump C"={"ASIA Pump #"=0, "channel"=0, "Simulated"=FALSE}, "FLOM Settings"={"VISA resource name"="", "Simulated?"=TRUE, "Pump Number"=0.0}, "SSI PR/LD Settings"={"VISA resource name"="", "Simulated?"=FALSE}, "SSI P40 Settings"={"VISA resource name"="", "Simulated?"=FALSE}, "Masterflex 75211 Settings"={"Analog DAQ Task"="", "Digital DAQ Task"=""}, "Pump Calibration File"=path "", "Calibration Slope"=0.0, "Calibration Y Intercept"=0.0, "Pump Cal Enum"=0}  # Configuration
            # "New settings are available, update the current ones stored in the shift register with the settings sent as part of the message"
            n120 = Variant To Data(error in=w364, type=w363, Variant=w365) -> (data=w358:T12, error out=w360:errorcluster)
            n121 = Bundle By Name(cluster=w361, "Configuration"=w358) -> (w359:T11)
          }
          frame "Exit" {
            # "Release the Logging queue reference"
            # "Don't check the error out. The UI message queue may have already been released."
            # "Stop the VI"
            # "Exit - Send the Exit message to the UI Message Handler.  Call 'Flush Data to Log File.vi' so any pending data is not lost."
            n122 = Release Queue(queue=w370, error in (no error)=w373) -> (error out=w369:errorcluster)  [unwired: 1 in, 2 out]
            n123 = call-poly "Enqueue Message.vi"("Priority Message? (F)"=TRUE, "Message"="Exit", "Message Queue"=w374) -> ("error out"=w368:errorcluster)  [unwired: 7 in, 1 out]
            n124 = call <vilib>:"Clear Errors.vi"("error in (no error)"=w368) -> ()  [unwired: 5 in, 2 out]
            n125 = Merge Errors(w369) -> (w375:errorcluster)
          }
          frame "---Copy This Frame---" {
            # "Duplicate this frame when creating new messages.  Change this comment in the duplicated frame to describe this message."
            n126 = Merge Errors(w380) -> (w379:errorcluster)
          }
          frame "In Error" {
            # "If we have a disconnect Error we will go to this state, and attempt to reconnect and get back to the pre-error state"
            n127 = Merge Errors(w399) -> (w396:errorcluster)
            n128 = call "Initialize.vi"("error in (no error)"=w396, "State in"=w398) -> ("error out"=w382:errorcluster, "Initialized"=w397:bool, "State out"=w393:T11)  [unwired: 7 in]
            n129 = Unbundle By Name(w393) -> ("Pump On?"=w386:enum16{"Off", "On", "Not Initialized"}, "Configuration.Cycle Period"=w387:dbl, "Data.Pump Speed"=w388:dbl, "Data.Pump Pressure"=w389:dbl, "Data.Pump Flow"=w390:dbl, "Configuration.Output Device"=w391:T3)
            n130 = Bundle By Name(cluster=w392, "Pump On?"=w386, "Cycle Period"=w387, "Current Pump Speed"=w388, "Current Pump Pressure"=w389, "Current Pump Flow"=w390, "Output"=w391) -> (w383:T2)
            n131 = call "Update if Clear.vi"("error in (no error)"=w382, "Message Data"=w383, "Queue in"=w384) -> ("error out"=w381:errorcluster)  [unwired: 8 in]
            n132 = case shown="False" w397 {
              tunnel: w385 -> [w404 w408]
              tunnel: w381 -> [w403 w407]
              tunnel: [w401 w410] -> w395
              tunnel: w393 -> [w401 w410]
              tunnel: [w400 w406] -> w394
              frame False {
                n133 = Wait (ms)(milliseconds to wait=u32 5000) -> ()  [unwired: 1 out]
                n134 = call-poly "Enqueue Message.vi"("error in (no error)"=w403, "Message"="In Error", "Message Queue"=w404) -> ("error out"=w400:errorcluster)  [unwired: 7 in, 1 out]
              }
              frame True {
                n135 = call-poly "Enqueue Message.vi"("error in (no error)"=w407, "Message"="Measure", "Message Queue"=w408) -> ("error out"=w406:errorcluster)  [unwired: 7 in, 1 out]
              }
            }
          }
          frame "Initialize" {
            # "Duplicate this frame when creating new messages.  Change this comment in the duplicated frame to describe this message."
            n136 = Merge Errors(w417) -> (w416:errorcluster)
            n137 = Bundle By Name(cluster=w414, "Log Started"=FALSE, "First Iteration"=TRUE) -> (w412:T11)
          }
          frame Default {
            # "'Default' case only runs if there is a message that isn't defined in any of the other cases.  Output a programming error."
            n138 = Concatenate Strings("The invalid message string " ("string"), w419, " was received in the Pump Module Engine." ("string")) -> (w420:string)
            n139 = Bundle By Name(cluster=errorcluster {"status"=TRUE, "code"=1, "source"=""} ("error constant"), "source"=w420) -> (w418:errorcluster)
          }
        }
        n140 = Unbundle By Name(w17) -> ("State"=w28:T10, "Configuration.Cycle Period"=w26:dbl)
        n141 = call "Error Handler.vi"("error in (no error)"=w34, "Message Queue"=w32) -> ("dup error in"=w33:errorcluster)  [unwired: 8 in, 1 out]
        n142 = case shown="\"Paused\"" w28 {
          tunnel: [w42 1 1] -> w27
          tunnel: w26 -> [w42 _ _]
          frame "Measuring" {
          }
          frame "Idle" {
          }
          frame "Paused" {
          }
        }
        n143 = node-c288(w27) -> ()  [unwired: 1 in, 1 out]
      }
      n144 = node-c288(w12) -> ()  [unwired: 1 out]
    }
    frame Error {
    }
  }
  "error out" <- w3
